vi "Make New Stage Limits File.vi"() -> ()   [LabVIEW 2020]
uses:
  Stages Limits Type Defs/Stages Limits Device Info and Limits.ctl
  Stages Limits Type Defs/Stage Limits.ctl
  Hardware Configuration/Hardware Configuration Controls/Device Type.ctl
panel:
  in  "Cancel":bool
  in  "Done":bool
  in  "Edit File":bool
  in  "Make New":bool
  in  "Device Limits Array":T1[](array[typedef])
  # "Click here to start a new file and overwrite any existing limits file."
  # "Click here to edit the current stage limits file."
  # "Use the horizontal scroll bar to change between stages."
  # "Axis No."
  # "Lower Limit (µm)"
  # "Upper Limit (µm)"
  # "1"
  # "2"
  # "3"
  # "4"
  # "5"
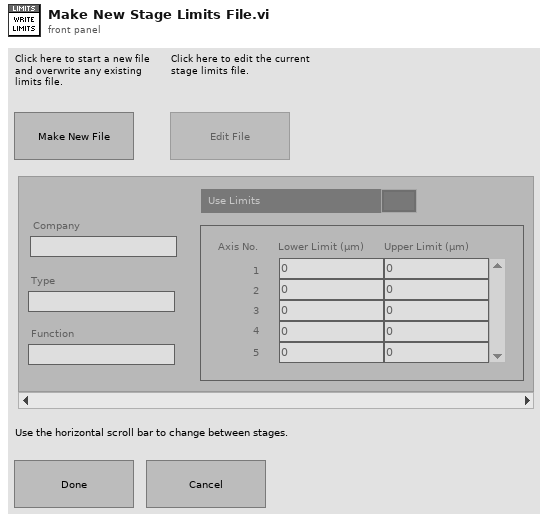
[diagram p1: front panel]
types:
  T1 = typedef "Stages Limits Device Info and Limits.ctl" = cluster{"Company":string, "Type":string, "Function":string, "Axis Limits":dbl[][], "Use Limits":bool}
  T2 = enum8{"Enabled", "Disabled", "Disabled and Grayed Out"}
  T3 = typedef "Stage Limits.ctl" = cluster{"Notifier":string, "Use Limits":bool, "Limits":dbl[][]}
  T4 = typedef "Device Type.ctl" = enum16{"AOTF", "Camera", "Deformable Mirror", "Laser", "Microscope Base", "Shutter", "Stage", "Waveform", "FPGA", "Email", "Filter Wheel", "Spinning Disk"}
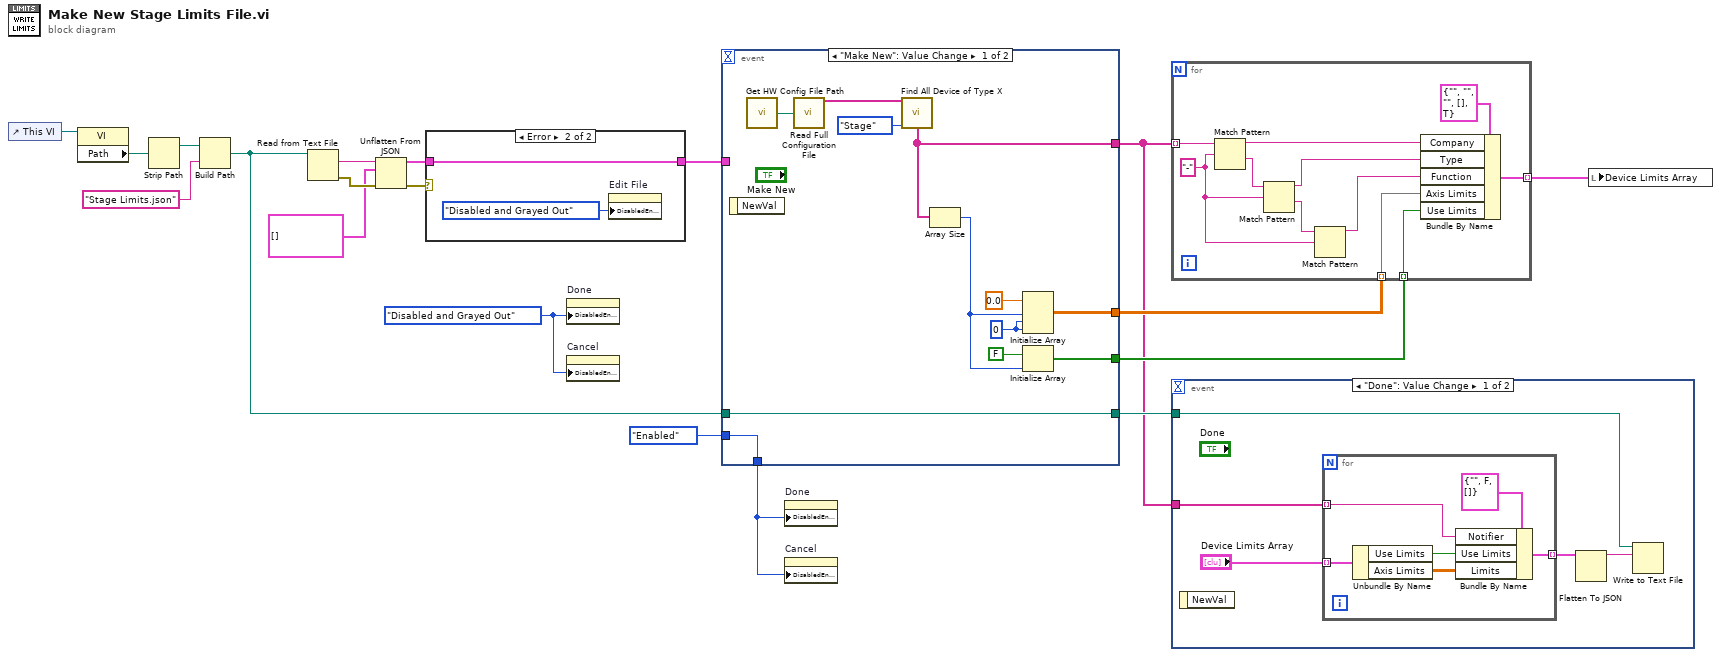
[diagram p0: block diagram]
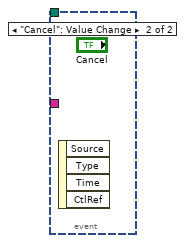
[diagram p2: hidden frame]
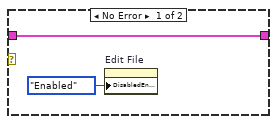
[diagram p3: hidden frame]
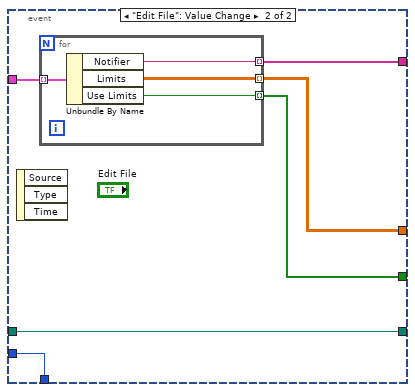
[diagram p4: hidden frame]
diagram:
  w3 = T2."Disabled and Grayed Out" ("Disabled")
  n1 = control-ref of="This VI"() -> (w19:refnum<vi>)
  n2 = property class="VI"(reference=w19) -> ("Path"=w18:path)  [unwired: 1 in, 2 out]
  n3 = Strip Path(path=w18) -> (stripped path=w17:path)  [unwired: 1 out]
  n4 = Build Path(base path=w17, name or relative path="Stage Limits.json") -> (appended path=w10:path)
  n5 = Read from Text File(file (use dialog)=w10) -> (text=w15:string, error out=w14:errorcluster)  [unwired: 3 in, 2 out]
  n6 = Unflatten From JSON(JSON string=w15, type and defaults=T3[] [], error in (no error)=w14) -> (value=w12:T3[], error out=w13:errorcluster)  [unwired: 4 in]
  n7 = case shown="Error" w13 {
    tunnel: w12 -> [w21 w22]
    tunnel: [w21 w22] -> w11
    frame No Error {
      n8 = property on="Edit File" class="Bool"("DisabledEnum"=T2."Enabled" ("Disabled")) -> ()  [unwired: 2 in, 2 out]
    }
    frame Error {
      n9 = property on="Edit File" class="Bool"("DisabledEnum"=T2."Disabled and Grayed Out" ("Disabled")) -> ()  [unwired: 2 in, 2 out]
    }
  }
  n10 = property on="Done" class="Bool"("DisabledEnum"=w3) -> ()  [unwired: 2 in, 2 out]
  n11 = property on="Cancel" class="Bool"("DisabledEnum"=w3) -> ()  [unwired: 2 in, 2 out]
  n12 = event shown="[0] \"Make New\": Value Change" {
    selector: _ -> [_ _]
    dyn-events: _ -> [_ _]
    timeout: _ -> [_ _]
    tunnel: w11 -> [_ w41]
    tunnel: w10 -> [w27 w37]
    tunnel: [w31 w40] -> w4
    tunnel: [w28 w38] -> w7
    tunnel: [w29 w39] -> w6
    tunnel: [w27 w37] -> w5
    tunnel: [w24 w36] -> w1
    tunnel: T2."Enabled" ("Disabled") -> [w24 w36]
    event "Make New": Value Change {
      w25 = 0 ("dimension size")
      n13 = event-data() -> ()  [unwired: 1 in, 1 out]
      n14 = call "Get HW Config File Path.vi"() -> ("File Path"=w33:path)  [unwired: 14 in, 1 out]
      n15 = call "Read Full Configuration File.vi"("Config File Path"=w33) -> ("Unique Notifier Names"=w34:string[])  [unwired: 11 in, 3 out]
      n16 = call "Find All Device of Type X.vi"("Unique Notifier Names"=w34, "Device Type"=Device_Type."Stage") -> ("All Devices"=w31:string[])  [unwired: 12 in, 1 out]
      n17 = Array Size(array=w31) -> (size(s)=w26:i32)
      n18 = Initialize Array(0.0 ("element"), w26, w25, w25) -> (w28:dbl[][][])
      n19 = Initialize Array(FALSE, w26) -> (w29:bool[])
    }
    event "Edit File": Value Change {
      n20 = event-data() -> ()  [unwired: 1 in, 3 out]
      n21 = for {
        tunnel: w41 -> [w45] mode=indexing
        tunnel: [w44] -> w40 mode=indexing
        tunnel: [w43] -> w39 mode=indexing
        tunnel: [w42] -> w38 mode=indexing
        n22 = Unbundle By Name(w45) -> ("Notifier"=w44:string, "Limits"=w42:dbl[][], "Use Limits"=w43:bool)
      }
    }
  }
  n23 = property on="Done" class="Bool"("DisabledEnum"=w1) -> ()  [unwired: 2 in, 2 out]
  n24 = property on="Cancel" class="Bool"("DisabledEnum"=w1) -> ()  [unwired: 2 in, 2 out]
  n25 = for {
    tunnel: w4 -> [w56] mode=indexing
    tunnel: w7 -> [w51] mode=indexing
    tunnel: [w50] -> w8 mode=indexing
    tunnel: w6 -> [w46] mode=indexing
    w48 = "-"
    n26 = Match Pattern(string=w56, regular expression=w48) -> (before substring=w53:string, after substring=w55:string)  [unwired: 1 in, 2 out]
    n27 = Match Pattern(string=w55, regular expression=w48) -> (before substring=w52:string, after substring=w49:string)  [unwired: 1 in, 2 out]
    n28 = Match Pattern(string=w49, regular expression=w48) -> (before substring=w47:string)  [unwired: 1 in, 3 out]
    n29 = Bundle By Name(cluster=T1 {"Company"="", "Type"="", "Function"="", "Axis Limits"=[], "Use Limits"=TRUE} ("Info and Limits"), "Company"=w53, "Type"=w52, "Function"=w47, "Axis Limits"=w51, "Use Limits"=w46) -> (w50:T1)
  }
  n30 = event shown="[0] \"Done\": Value Change" {
    selector: _ -> [_ _]
    dyn-events: _ -> [_ _]
    timeout: _ -> [_ _]
    tunnel: w5 -> [w58 _]
    tunnel: w4 -> [w57 _]
    event "Done": Value Change {
      n31 = event-data() -> ()  [unwired: 1 in, 1 out]
      n32 = for {
        tunnel: "Device Limits Array" -> [w67] mode=indexing
        tunnel: [w63] -> w59 mode=indexing
        tunnel: w57 -> [w62] mode=indexing
        n33 = Unbundle By Name(w67) -> ("Use Limits"=w65:bool, "Axis Limits"=w64:dbl[][])
        n34 = Bundle By Name(cluster=T3 {"Notifier"="", "Use Limits"=FALSE, "Limits"=[]} ("Stage Limits"), "Notifier"=w62, "Use Limits"=w65, "Limits"=w64) -> (w63:T3)
      }
      n35 = Flatten To JSON(anything=w59) -> (JSON string=w61:string)  [unwired: 2 in, 1 out]
      n36 = Write to Text File(file (use dialog)=w58, text=w61) -> ()  [unwired: 2 in, 3 out]
    }
    event "Cancel": Value Change {
      n37 = event-data() -> ()  [unwired: 1 in, 4 out]
    }
  }
  n38 = local write "Device Limits Array"(w8) -> ()
